vi "KH_DAQ_TURCK_Global.vi"() -> ()   [LabVIEW 2021]
panel:
  out "NamesDO":string[](array[string])
  out "Anzahl_DXP_DXP":i32
  out "NamesDI":string[](array[string])
  out "Anzahl_DO_RFID":i32
  out "Anzahl_DO_IOL":i32
  out "Anzahl_DO_DXP":i32
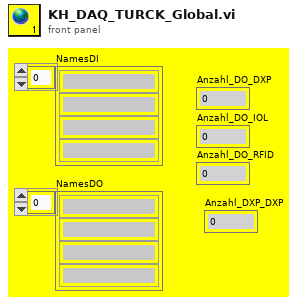
[diagram p1: front panel]
diagram:
